vi "LastWeekCheck(SubVI).vi"(11 "List of Weeks":u8[](array[numeric])) -> (3 "Array":u8[](array[numeric]))   [LabVIEW 2017, in "DS_Lib.lvlib" / "SRReportParser.lvlib"]
doc: "Checks whether to include or not the last week from the weeks arrays. It is based on the current week number and weekday"
uses:
  SRReportParser.lvlib
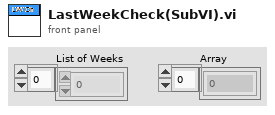
[diagram p1: front panel]
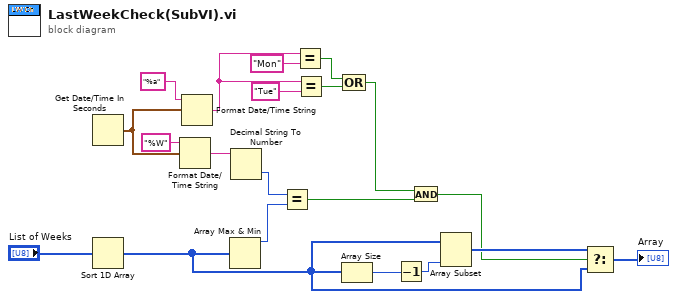
[diagram p0: block diagram]
diagram:
  n1 = Get Date/Time In Seconds() -> (seconds since 1Jan1904=w2:timestamp)
  n2 = Sort 1D Array(array="List of Weeks") -> (sorted array=w19:u8[])
  n3 = Format Date/Time String(time format string (%c)="%W", seconds (now)=w2) -> (date/time string=w5:string)  [unwired: 1 in]
  n4 = Format Date/Time String(time format string (%c)="%a", seconds (now)=w2) -> (date/time string=w11:string)  [unwired: 1 in]
  n5 = Array Max & Min(array=w19) -> (max value=w7:u8)  [unwired: 3 out]
  n6 = Decimal String To Number(string=w5) -> (number=w6:i32)  [unwired: 2 in, 1 out]
  n7 = Equal?(x=w6, y=w7) -> (x = y?=w8:bool)
  n8 = Equal?(x=w11, y="Mon") -> (x = y?=w12:bool)
  n9 = Equal?(x=w11, y="Tue") -> (x = y?=w13:bool)
  n10 = Array Size(array=w19) -> (size(s)=w15:i32)
  n11 = Compound Arithmetic op=OR(w12, w13) -> (w14:bool)
  n12 = Decrement(x=w15) -> (x-1=w16:i32)
  n13 = And(x=w14, y=w8) -> (x .and. y?=w17:bool)
  n14 = Array Subset(array=w19, length=w16) -> (w18:u8[])  [unwired: 1 in]
  n15 = Select(t=w18, s=w17, f=w19) -> (s? t:f=→"Array":u8[])
